vi "Page_Info_Write.vi"(6 "ctlReferences":T1, 8 "error in (no error)":errorcluster, 10 "Target filename":string, 11 "AB_InteropAssembly in":refnum<class "AB_InteropAssembly.lvclass">) -> (0 "error out":errorcluster, 3 "AB_InteropAssembly out":refnum<class "AB_InteropAssembly.lvclass">)   [LabVIEW 2020, in "AB_InteropAssembly.lvclass"]
uses:
  <vilib>/AppBuilder/AB_Classes/InteropAssembly/AB_InteropAssembly.lvclass
  <resource>/Framework/Providers/Builds/AppBuilder/AB_UI_Page_Info_References.ctl
  <vilib>/AppBuilder/AB_Classes/InteropAssembly/AB_InteropAssembly.lvclass/AB_InteropAssembly.ctl
  <vilib>/AppBuilder/AB_Classes/Application/AB_Application.lvclass
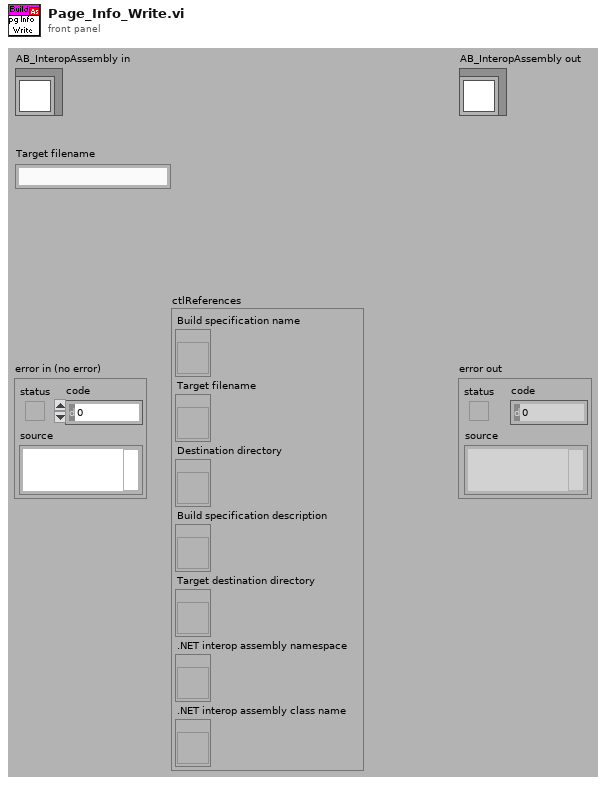
[diagram p1: front panel]
types:
  T1 = typedef "AB_UI_Page_Info_References.ctl" = cluster{"Build specification name":refnum<vi>, "Target filename":refnum<vi>, "Destination directory":refnum<vi>, "Build specification description":refnum<vi>, "Target destination directory":refnum<vi>, ".NET interop assembly namespace":refnum<vi>, ".NET interop assembly class name":refnum<vi>}
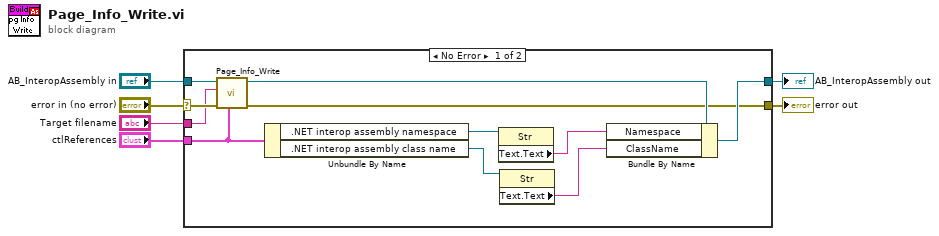
[diagram p0: block diagram]
diagram:
  n1 = case shown="No Error" "error in (no error)" {
    selector: "error in (no error)" -> [w9 w19]
    tunnel: [w8 w19] -> w5
    tunnel: [w10 w18] -> w3
    tunnel: "AB_InteropAssembly in" -> [w17 w18]
    tunnel: "ctlReferences" -> [w16 _]
    tunnel: "Target filename" -> [w7 _]
    frame No Error {
      n2 = call-parent "Page_Info_Write.vi"("ctlReferences"=w16, "error in (no error)"=w9, "Target filename"=w7, "AB_Targetfile in"=w17) -> ("error out"=w8:errorcluster, "AB_Targetfile out"=w15:refnum<class "AB_InteropAssembly.lvclass">)  [unwired: 6 out]
      n3 = Unbundle By Name(w16) -> (".NET interop assembly namespace"=w14:refnum<vi>, ".NET interop assembly class name"=w12:refnum<vi>)
      n4 = property class="Str"(reference=w14) -> ("Text.Text"=w13:string)  [unwired: 1 in, 2 out]
      n5 = property class="Str"(reference=w12) -> ("Text.Text"=w11:string)  [unwired: 1 in, 2 out]
      n6 = Bundle By Name(cluster=w15, "Namespace"=w13, "ClassName"=w11) -> (w10:refnum<class "AB_InteropAssembly.lvclass">)
    }
    frame Error {
    }
  }
  "error out" <- w5
  "AB_InteropAssembly out" <- w3
